vi "uintNotEqual.vi"(8 "Error in (no error)":errorcluster, 10 "Int2 in":refnum<class "UintClass.lvclass">, 11 "Int1 in":refnum<class "UintClass.lvclass">) -> (0 "Error out":errorcluster, 1 "Timing":u32, 3 "Int1 != Int2?":bool)   [LabVIEW 2011, in "UintClass.lvclass"]
uses:
  UintClass.lvclass
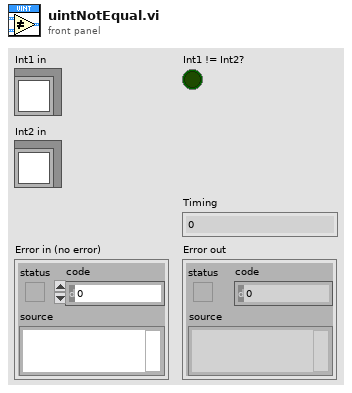
[diagram p1: front panel]
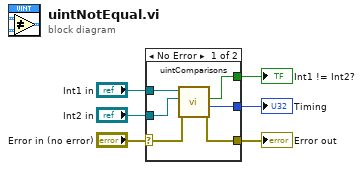
[diagram p0: block diagram]
diagram:
  n1 = case shown="No Error" "Error in (no error)" {
    selector: "Error in (no error)" -> [w10 w13]
    tunnel: [w9 w13] -> w5
    tunnel: "Int1 in" -> [w12 _]
    tunnel: "Int2 in" -> [w11 _]
    tunnel: [w8 _] -> w2
    tunnel: [w7 _] -> w1
    frame No Error {
      n2 = call "uintComparisons.vi"("Error in (no error)"=w10, "Int2 in"=w11, "Int1 in"=w12) -> ("Error out"=w9:errorcluster, "Timing"=w8:u32, "Uint1 != Uint2?"=w7:bool)  [unwired: 1 in, 5 out]
    }
    frame Error {
    }
  }
  "Error out" <- w5
  "Timing" <- w2
  "Int1 != Int2?" <- w1
